vi "GetEmbeddedName.vi"(6 "timeout in ms (-1)":i32=-1, 8 "error in (no error)":errorcluster, 11 "EmbeddedSMO in":refnum<class "EmbeddedSMO.lvclass">) -> (0 "error out":errorcluster, 2 "Name":string, 3 "EmbeddedSMO out":refnum<class "EmbeddedSMO.lvclass">)   [LabVIEW 2016, in "EmbeddedSMO.lvclass"]
uses:
  EmbeddedSMO.lvclass
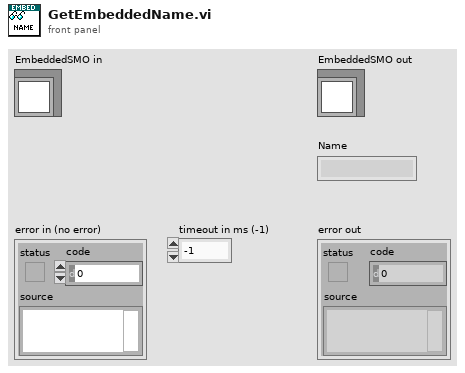
[diagram p1: front panel]
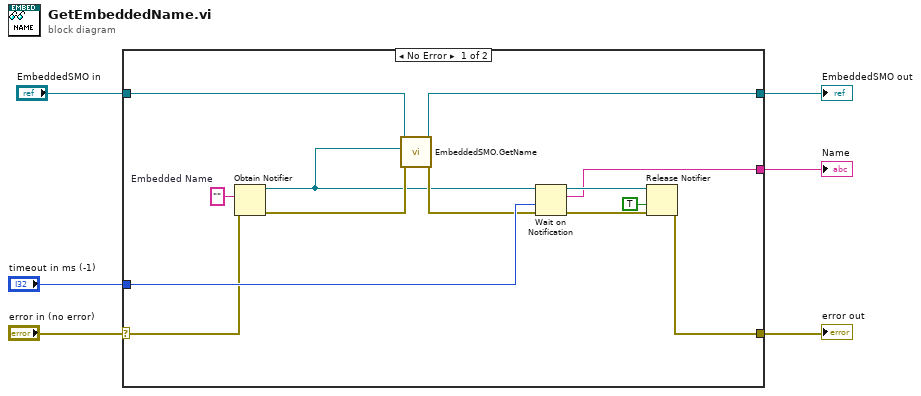
[diagram p0: block diagram]
diagram:
  n1 = case shown="No Error" "error in (no error)" {
    selector: "error in (no error)" -> [w14 w21]
    tunnel: [w13 w21] -> w5
    tunnel: [w7 w20] -> w4
    tunnel: "EmbeddedSMO in" -> [w8 w20]
    tunnel: [w17 _] -> w2
    tunnel: "timeout in ms (-1)" -> [w15 _]
    frame No Error {
      w12 = ""  # Embedded Name
      n2 = Obtain Notifier(notification data type=w12, error in (no error)=w14) -> (notifier out=w9:refnum<notifier>, error out=w11:errorcluster)  [unwired: 2 in, 1 out]
      n3 = call "EmbeddedSMO.GetName.vi"("error in (no error)"=w11, "GetName"=w9, "EmbeddedSMO"=w8) -> ("error out"=w10:errorcluster, "EmbeddedSMO out"=w7:refnum<class "EmbeddedSMO.lvclass">)  [unwired: 7 in]
      n4 = Wait on Notification(notifier=w9, timeout in ms (-1)=w15, error in (no error)=w10) -> (notifier out=w19:refnum<notifier>, notification=w17:string, error out=w16:errorcluster)  [unwired: 1 in, 1 out]
      n5 = Release Notifier(notifier=w19, force destroy? (F)=TRUE, error in (no error)=w16) -> (error out=w13:errorcluster)  [unwired: 2 out]
    }
    frame Error {
    }
  }
  "error out" <- w5
  "EmbeddedSMO out" <- w4
  "Name" <- w2
